vi "Select_User.vi"() -> ()   [LabVIEW 2016]
uses:
  <vilib>/Utility/miscctls.llb/LVPointTypeDef.ctl
  <vilib>/Utility/config.llb/NI_LVConfig.lvlib
panel:
  out "Controls references":T1
  out "GoToTracker indicator for Latching inside Events workaround":bool
  out "TestComm indicator for Latching inside Events workaround":bool
  in  "Login tab":enum32{"Login", "Settings", "Manage users"}(tab)
  in  "Go to Tracker":bool
  in  "Select User":u16(ring) items=["Admin"]
  in  "Enter password":string
  in  "Jump to tracking":bool
  in  "Button cover":bool
  out "Comm. test results":bool
  in  "Test VISA Comms":bool
  in  "VISA":refnum<visa-resource-name>="Tracker"
  in  "Cancel Users Update":bool
  in  "Save Users":bool
  in  "... or add new one":string
  in  "Reset or create password":string
  in  "Select User for update":u16(ring) items=["Admin"]
  in  "Delete current user":bool
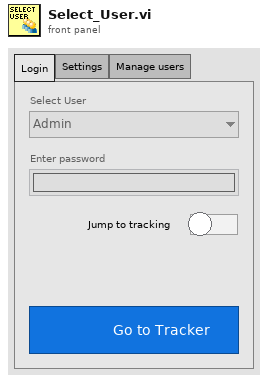
[diagram p1: front panel]
types:
  T1 = cluster{"Tabs":refnum<vi>, "Select User at login page":refnum<vi>, "Enter password":refnum<vi>, "Jump to tracking":refnum<vi>, "Test VISA Comms button":refnum<vi>, "Comm. test results indicator":refnum<vi>, "Select User for update":refnum<vi>, "Go to Tracker":refnum<vi>, "Jump to tracking":refnum<vi>, "... or add new one":refnum<vi>, "Reset or create password":refnum<vi>, "Delete current user":refnum<vi>}
  T2 = enum8{"Enabled", "Disabled", "Disabled and Grayed Out"}
  T3 = cluster{"Numeric Control":u32, "Numeric Control":u32}[]
  T4 = typedef "LVPointTypeDef.ctl" = cluster{"Horizontal":i16, "Vertical":i16}
  T5 = typedef "NI_LVConfig.lvlib/Config Data RefNum.ctl" = refnum<k1>
  T6 = typedef "eventvkey.ctl" = enum16{"ASCII", "Enter", "Return", "Shift", "Ctrl", "Alt", "Cmd", "Opt", "Caps", "NumLock", "Clear", "Break", "Up", "Down", "Left", "Right", "Insert", "Delete", "Home", "End", "PageUp", "PageDown", "Escape", "Help", "Pause", "ScrollLock", "F1", "F2", "F3", "F4", "F5", "F6", "F7", "F8", "F9", "F10", "F11", "F12", "F13", "F14", "F15", "F16", "F17", "F18", "F19", "F20", "F21", "F22", "F23", "F24", "Play", "VolumeUp", "VolumeDown", "Mute", "Two Byte Char"}
  T7 = enum32{"Page Enabled", "Page Disabled", "Page Disabled & Grayed"}
  T8 = cluster{"Data acquisition status":refnum<notifier>, "Play/Pause status":refnum<notifier>, "Complete stop":refnum<notifier>, "Temp file ready for processing":refnum<notifier>, "Has been recorded":refnum<notifier>, "Recording now":refnum<notifier>, "Path to the latest complete temp file":refnum<notifier>}
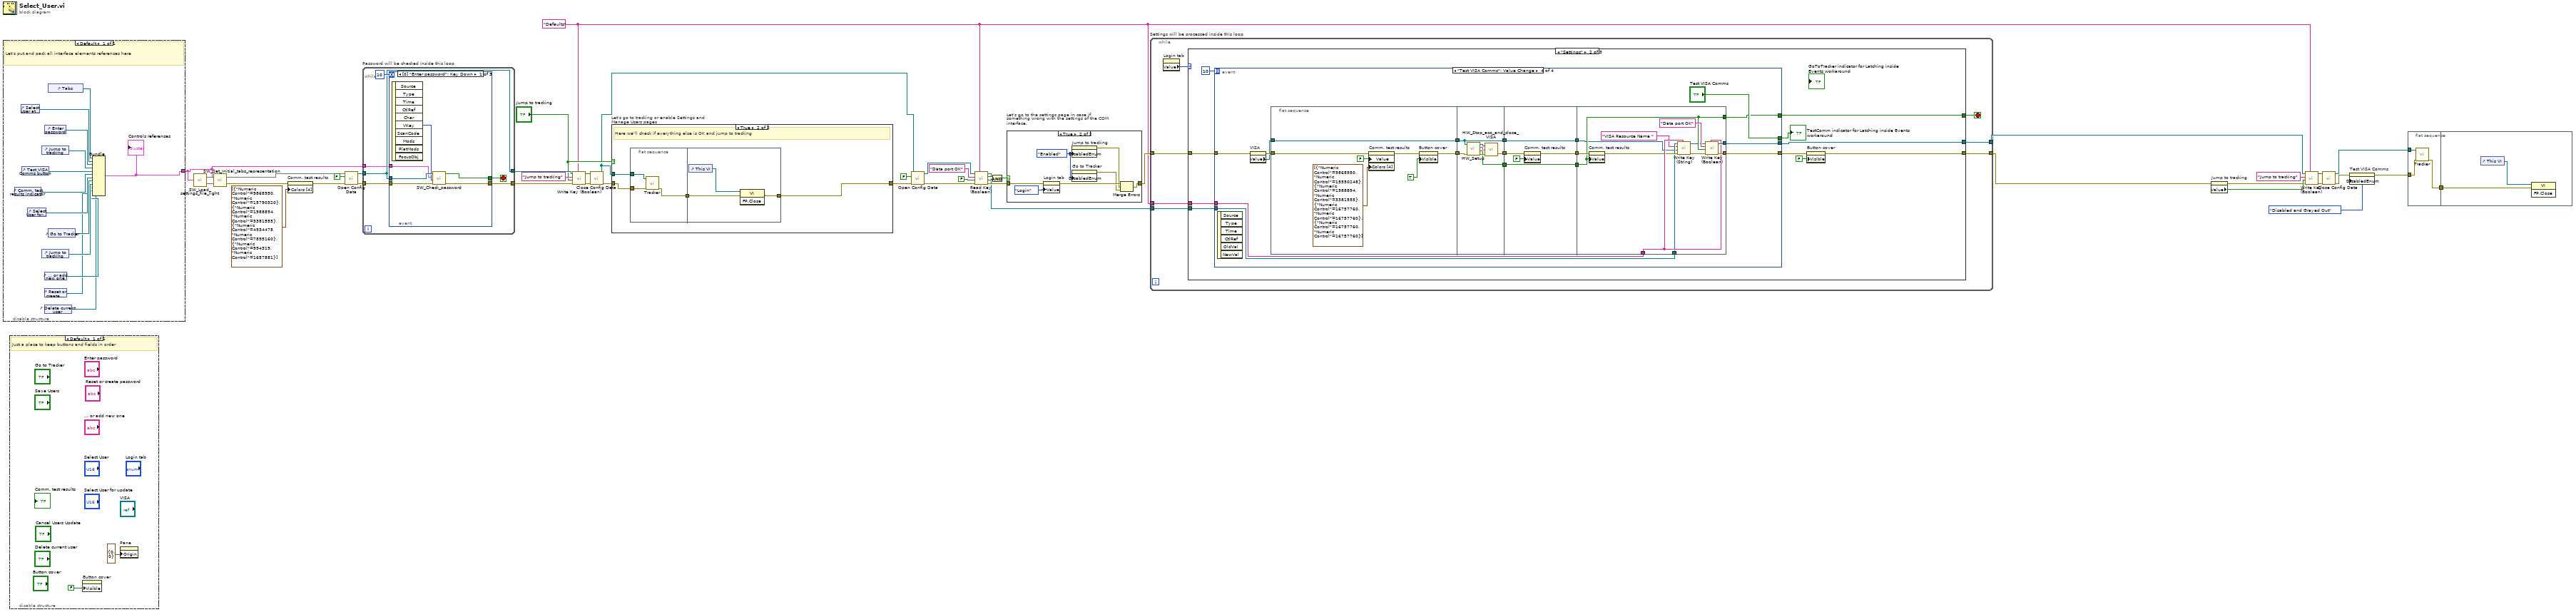
[diagram p0: block diagram]
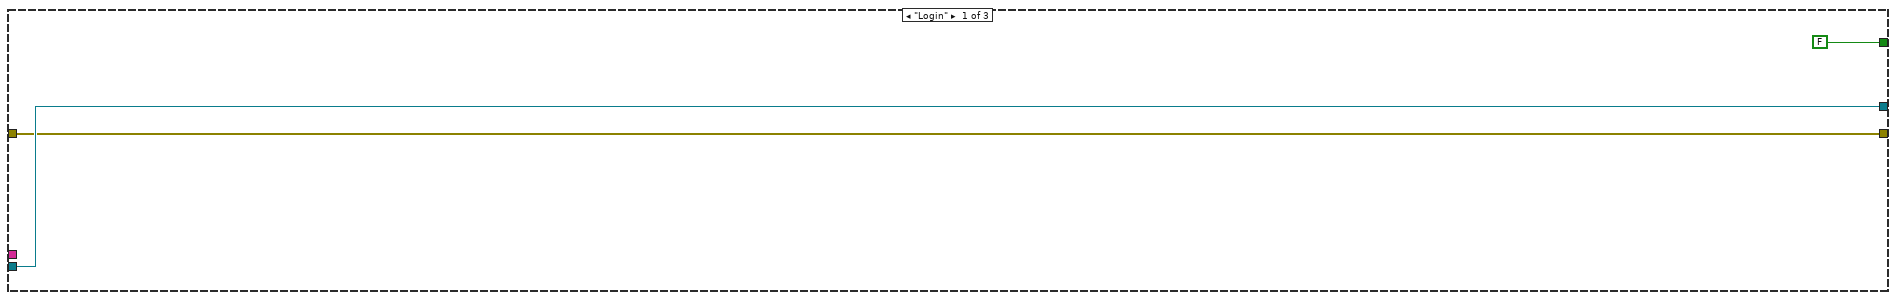
[diagram p2: hidden frame]
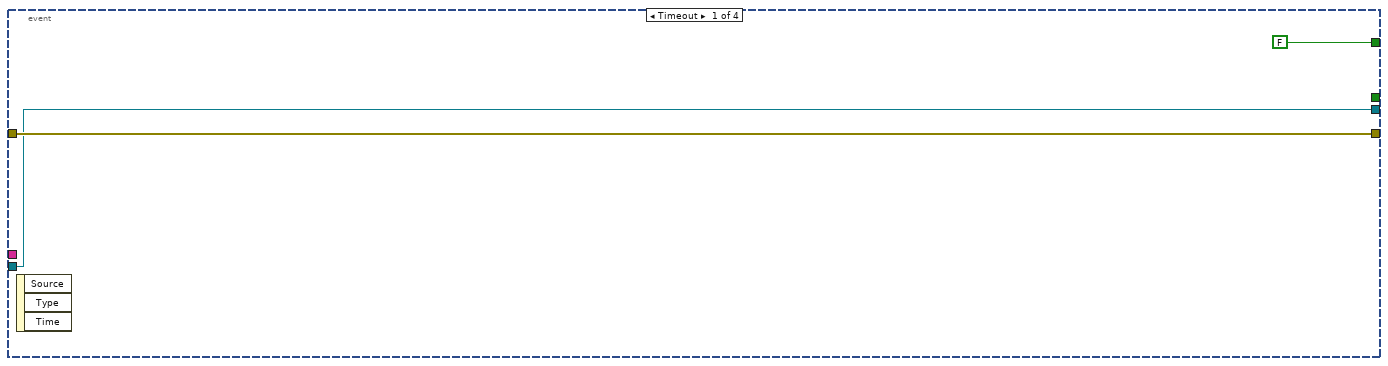
[diagram p3: hidden frame]
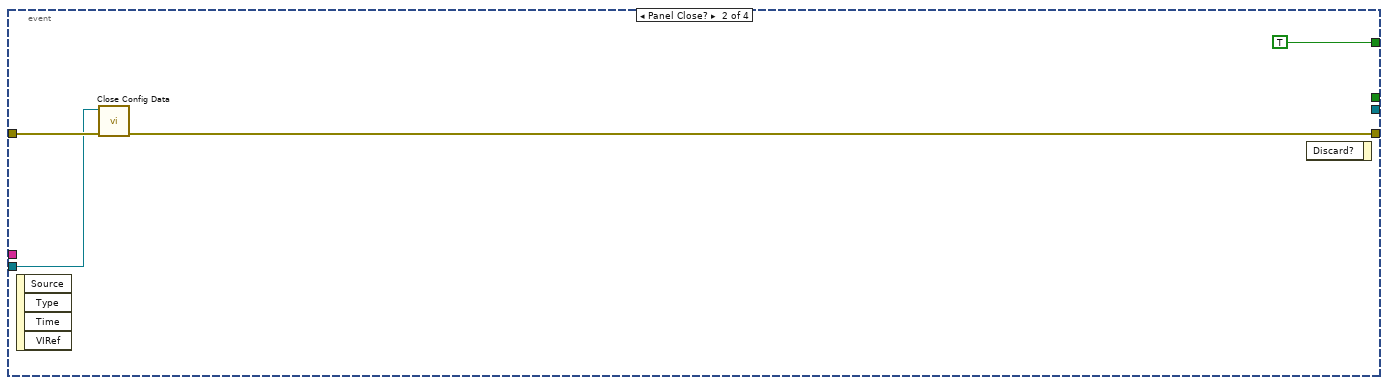
[diagram p4: hidden frame]
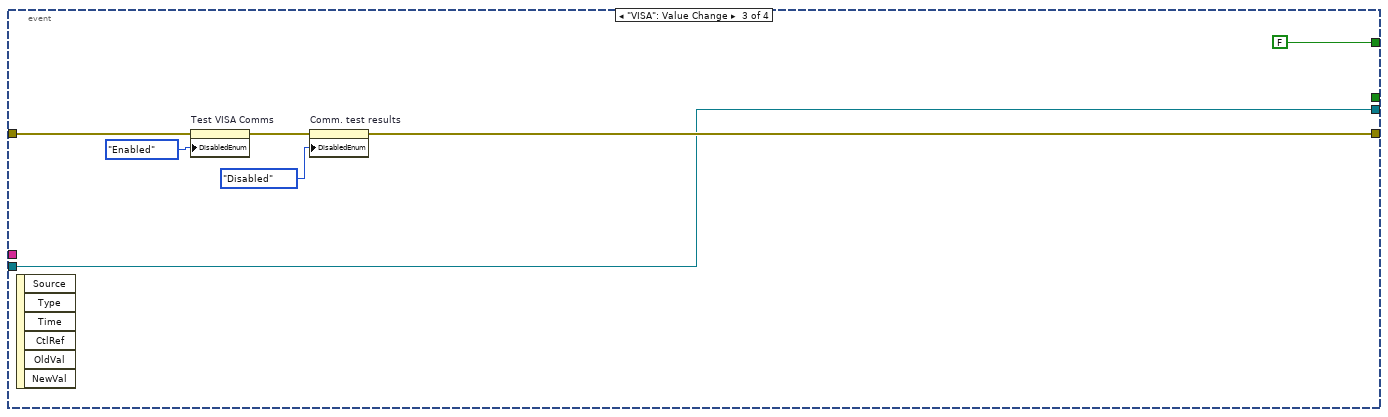
[diagram p5: hidden frame]
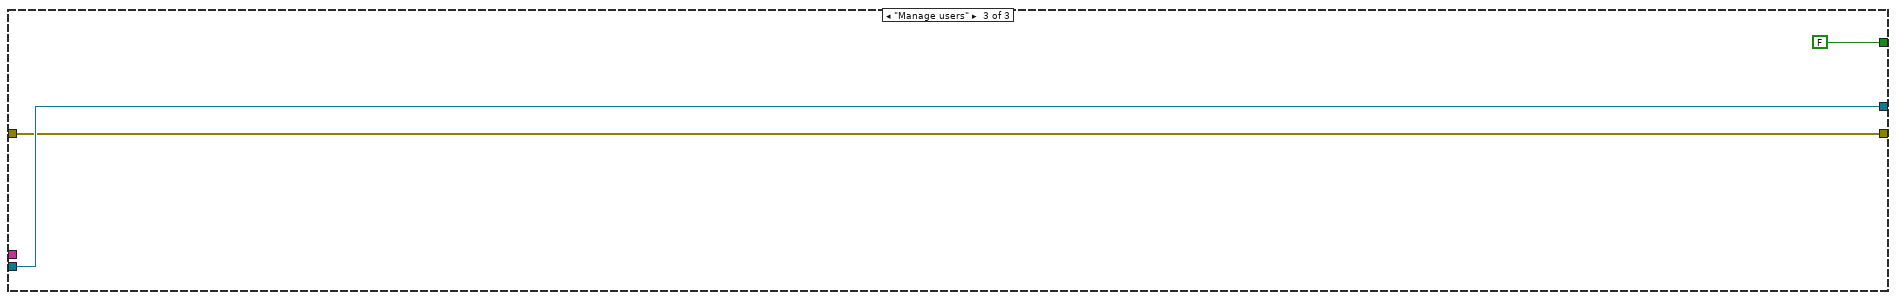
[diagram p6: hidden frame]
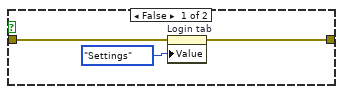
[diagram p7: hidden frame]
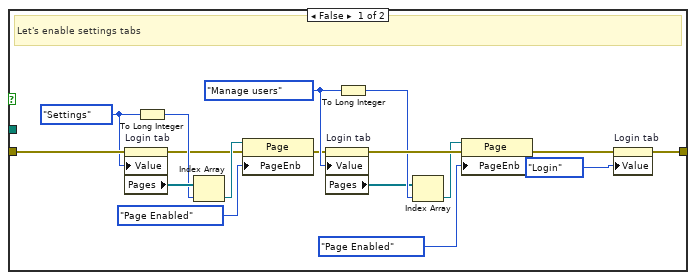
[diagram p8: hidden frame]
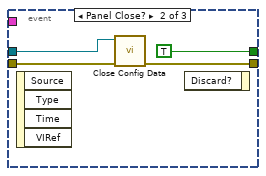
[diagram p9: hidden frame]
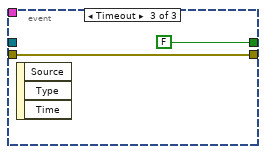
[diagram p10: hidden frame]
diagram:
  w9 = "Defaults" ("section")
  n1 = disable-structure "Conditional Disable Structure" shown="Default" {
    disable-tunnel: [w43] -> w3
    frame Enabled {
      # "Let's put and pack all interface elements references here"
      n2 = control-ref of="Comm. test results indicator"() -> (w50:refnum<vi>)
      n3 = control-ref of="Select User at login page"() -> (w54:refnum<vi>)
      n4 = control-ref of="Test VISA Comms button"() -> (w51:refnum<vi>)
      n5 = control-ref of="Select User for update"() -> (w49:refnum<vi>)
      n6 = control-ref of="Jump to tracking"() -> (w52:refnum<vi>)
      n7 = control-ref of="Jump to tracking"() -> (w47:refnum<vi>)
      n8 = control-ref of="Enter password"() -> (w53:refnum<vi>)
      n9 = control-ref of="... or add new one"() -> (w46:refnum<vi>)
      n10 = control-ref of="Reset or create password"() -> (w45:refnum<vi>)
      n11 = control-ref of="Delete current user"() -> (w44:refnum<vi>)
      n12 = control-ref of="Tabs"() -> (w55:refnum<vi>)
      n13 = control-ref of="Go to Tracker"() -> (w48:refnum<vi>)
      n14 = Bundle("Tabs"=w55, "Select User at login page"=w54, "Enter password"=w53, "Jump to tracking"=w52, "Test VISA Comms button"=w51, "Comm. test results indicator"=w50, "Select User for update"=w49, "Go to Tracker"=w48, "Jump to tracking"=w47, "... or add new one"=w46, "Reset or create password"=w45, "Delete current user"=w44) -> (w43:T1)  [unwired: 1 in]
      "Controls references" <- w43
    }
  }
  n15 = disable-structure shown="Default" {
    frame Enabled {
      # "Just a place to keep buttons and fields in order"
      n16 = property on="Button cover" class="Bool"("Visible"=FALSE) -> ()  [unwired: 2 in, 2 out]
      n17 = property on="Pane" class="Pane"("Origin"=T4 {"Horizontal"=0, "Vertical"=0}) -> ()  [unwired: 2 in, 2 out]
    }
  }
  n18 = call "SW_Load_settings_file_light.vi"(0:w3) -> (1:w22, 2:w40)
  n19 = call "SW_Set_Initial_tabs_representation.vi"("error in (no error)"=w40, "Controls references"=w3) -> ("error out"=w18:errorcluster)  [unwired: 1 in]
  n20 = property on="Comm. test results" class="Bool (strict)"(error in=w18, "Colors [4]"=T3 [{"Numeric Control"=9868950, "Numeric Control"=15790320}, {"Numeric Control"=1988894, "Numeric Control"=3381555}, {"Numeric Control"=4934475, "Numeric Control"=7895160}, {"Numeric Control"=994319, "Numeric Control"=1657881}]) -> (error out=w19:errorcluster)  [unwired: 1 in, 1 out]
  n21 = call <vilib>:"Open Config Data.vi"("error in (no error)"=w19, "create file if necessary (T)"=FALSE, "configuration file path"=w22) -> ("error out"=w41:errorcluster, "refnum"=w42:T5)  [unwired: 6 in, 1 out]
  n22 = while "Password will be checked inside this loop" {
    tunnel: w41 -> [w62]
    tunnel: w42 -> [w60]
    tunnel: [w61] -> w38
    tunnel: [w60] -> w39
    tunnel: w3 -> [w58]
    stop <- w59 stop-if-true
    n23 = event shown="[0] \"Enter password\": Key Down" {
      selector: _ -> [_ _ _]
      dyn-events: _ -> [_ _ _]
      timeout: 10 -> [_ _ _]
      tunnel: w62 -> [w69 w72 w74]
      tunnel: w60 -> [w68 w70 _]
      tunnel: [w66 TRUE ("Stop the loop") FALSE] -> w59
      tunnel: [w65 w71 w74] -> w61
      tunnel: w58 -> [w64 _ _]
      event "Enter password": Key Down {
        n24 = event-data() -> ("VKey"=w67:T6)  [unwired: 1 in, 9 out]
        n25 = call "SW_Check_password.vi"("error in (no error)"=w69, "Entered key"=w67, "Controls references"=w64, "Configuration file refnum in"=w68) -> ("error out"=w65:errorcluster, "Password OK"=w66:bool)  [unwired: 5 in, 1 out]
      }
      event Panel Close? {
        n26 = event-data() -> ()  [unwired: 1 in, 4 out]
        n27 = call <vilib>:"Close Config Data.vi"("error in (no error)"=w72, "refnum"=w70) -> ("error out"=w71:errorcluster)  [unwired: 8 in, 1 out]
        n28 = event-data() -> ()  [unwired: 2 in, 1 out]
      }
      event Timeout {
        n29 = event-data() -> ()  [unwired: 1 in, 3 out]
      }
    }
  }
  n30 = call <vilib>:"Write Key (Boolean).vi"("section"=w9, "error in (no error)"=w38, "value"="Jump to tracking", "key"="Jump to tracking", "refnum"=w39) -> ("error out"=w30:errorcluster, "refnum out"=w28:T5)  [unwired: 4 in, 1 out]
  n31 = call <vilib>:"Close Config Data.vi"("error in (no error)"=w30, "refnum"=w28) -> ("error out"=w29:errorcluster, "file path"=w1:path)  [unwired: 8 in]
  n32 = case "Let's go to tracking or enable Settings and Manage Users pages" shown="True" "Jump to tracking" {
    tunnel: w29 -> [w92 w96]
    tunnel: [w77 w93] -> w27
    tunnel: w1 -> [_ w95]
    frame False {
      w81 = enum32{"Login", "Settings", "Manage users"}."Manage users" ("Login tab")
      w90 = enum32{"Login", "Settings", "Manage users"}."Settings" ("Login tab")
      # "Let's enable settings tabs"
      n33 = property on="Login tab" class="TabCtl (strict)"(error in=w92, "Value"=w90) -> (error out=w87:errorcluster, "Pages"=w91:refnum<vi>[])  [unwired: 1 in, 1 out]
      n34 = To Long Integer(number=w90) -> (32bit integer=w89:i32)
      n35 = Index Array(array=w91, index=w89) -> (element=w88:refnum<vi>)
      n36 = property class="Page"(reference=w88, error in=w87, "PageEnb"=T7."Page Enabled" ("Page Enabled State")) -> (error out=w79:errorcluster)  [unwired: 1 out]
      n37 = property on="Login tab" class="TabCtl (strict)"(error in=w79, "Value"=w81) -> (error out=w84:errorcluster, "Pages"=w80:refnum<vi>[])  [unwired: 1 in, 1 out]
      n38 = To Long Integer(number=w81) -> (32bit integer=w82:i32)
      n39 = Index Array(array=w80, index=w82) -> (element=w83:refnum<vi>)
      n40 = property class="Page"(reference=w83, error in=w84, "PageEnb"=T7."Page Enabled" ("Page Enabled State")) -> (error out=w78:errorcluster)  [unwired: 1 out]
      n41 = property on="Login tab" class="TabCtl (strict)"(error in=w78, "Value"=enum32{"Login", "Settings", "Manage users"}."Login" ("Login tab")) -> (error out=w77:errorcluster)  [unwired: 1 in, 1 out]
    }
    frame True {
      # "Here we'll check if everything else is OK and jump to tracking"
      n42 = flat-sequence {
        tunnel: w96 -> [w99]
        tunnel: w95 -> [w98]
        tunnel: [w97] -> w94
        tunnel: w94 -> [w101]
        tunnel: [w100] -> w93
        frame #0 {
          n43 = call "Tracker.vi"("error in (no error)"=w99, "Settings file path"=w98) -> ("error out"=w97:errorcluster)  [unwired: 9 in]
        }
        frame #1 {
          n44 = control-ref of="This VI"() -> (w102:refnum<vi>)
          n45 = invoke class="VI" method="FP.Close"(reference=w102, error in=w101) -> (error out=w100:errorcluster)  [unwired: 1 in, 2 out]
        }
      }
    }
  }
  n46 = call <vilib>:"Open Config Data.vi"("error in (no error)"=w27, "create file if necessary (T)"=FALSE, "configuration file path"=w1) -> ("error out"=w26:errorcluster, "refnum"=w25:T5)  [unwired: 6 in, 1 out]
  n47 = call <vilib>:"Read Key (Boolean).vi"("section"=w9, "error in (no error)"=w26, "default value"=FALSE, "key"="Data port OK", "refnum"=w25) -> ("error out"=w31:errorcluster, "value"=w33:bool, "found?"=w34:bool, "refnum out"=w20:T5)  [unwired: 3 in]
  n48 = And(x=w34, y=w33) -> (x .and. y?=w32:bool)
  n49 = case "Let's go to the settings page in case if something wrong with the settings of the COM interface." shown="True" w32 {
    tunnel: w31 -> [w103 w112]
    tunnel: [w105 w109] -> w21
    frame False {
      n50 = property on="Login tab" class="TabCtl (strict)"(error in=w103, "Value"=enum32{"Login", "Settings", "Manage users"}."Settings" ("Login tab")) -> (error out=w105:errorcluster)  [unwired: 1 in, 1 out]
    }
    frame True {
      w110 = T2."Enabled" ("Disabled")
      n51 = property on="Login tab" class="TabCtl (strict)"(error in=w112, "Value"=enum32{"Login", "Settings", "Manage users"}."Login" ("Login tab")) -> (error out=w108:errorcluster)  [unwired: 1 in, 1 out]
      n52 = property on="Jump to tracking" class="Bool (strict)"("DisabledEnum"=w110) -> (error out=w107:errorcluster)  [unwired: 2 in, 1 out]
      n53 = property on="Go to Tracker" class="Bool"("DisabledEnum"=w110) -> (error out=w106:errorcluster)  [unwired: 2 in, 1 out]
      n54 = Merge Errors(w108, w107, w106) -> (w109:errorcluster)
    }
  }
  n55 = while "Settings will be processed inside this loop" {
    tunnel: w21 -> [w119]
    tunnel: w20 -> [w115]
    tunnel: [w117] -> w15
    tunnel: [w116] -> w14
    tunnel: w9 -> [w114]
    stop <- w118 stop-if-true
    n56 = property on="Login tab" class="TabCtl (strict)"() -> ("Value"=w113:enum32{"Login", "Settings", "Manage users"})  [unwired: 2 in, 2 out]
    n57 = case shown="\"Settings\"" w113 {
      tunnel: w119 -> [w121 w131 w196]
      tunnel: [FALSE ("Instrument OK?") w130 FALSE ("Instrument OK?")] -> w118
      tunnel: [w121 w126 w196] -> w117
      tunnel: [w122 w125 w197] -> w116
      tunnel: w115 -> [w122 w124 w197]
      tunnel: w114 -> [_ w123 _]
      frame "Login" {
      }
      frame "Settings" {
        n58 = event shown="[3] \"Test VISA Comms\": Value Change" {
          selector: _ -> [_ _ _ _]
          dyn-events: _ -> [_ _ _ _]
          timeout: 10 -> [_ _ _ _]
          tunnel: [w135 w137 w142 w158] -> w127
          tunnel: w131 -> [w135 w138 w146 w163]
          tunnel: [FALSE TRUE FALSE w149] -> w130
          tunnel: [_ _ _ "Test VISA Comms"] -> w129
          tunnel: [w133 _ w140 w151] -> w125
          tunnel: w124 -> [w133 w136 w140 w150]
          tunnel: w123 -> [_ _ _ w152]
          event Timeout {
            n59 = event-data() -> ()  [unwired: 1 in, 3 out]
          }
          event Panel Close? {
            n60 = event-data() -> ()  [unwired: 1 in, 4 out]
            n61 = call <vilib>:"Close Config Data.vi"("error in (no error)"=w138, "refnum"=w136) -> ("error out"=w137:errorcluster)  [unwired: 8 in, 1 out]
            n62 = event-data() -> ()  [unwired: 2 in, 1 out]
          }
          event "VISA": Value Change {
            n63 = event-data() -> ()  [unwired: 1 in, 6 out]
            n64 = property on="Test VISA Comms" class="Bool"(error in=w146, "DisabledEnum"=T2."Enabled" ("Disabled")) -> (error out=w145:errorcluster)  [unwired: 1 in, 1 out]
            n65 = property on="Comm. test results" class="Bool (strict)"(error in=w145, "DisabledEnum"=T2."Disabled" ("Disabled")) -> (error out=w142:errorcluster)  [unwired: 1 in, 1 out]
          }
          event "Test VISA Comms": Value Change {
            n66 = event-data() -> ()  [unwired: 1 in, 6 out]
            n67 = property on="VISA" class="VISAName"(error in=w163) -> (error out=w162:errorcluster, "Value"=w161:refnum<visa-resource-name>)  [unwired: 1 in, 1 out]
            n68 = flat-sequence {
              tunnel: w162 -> [w168]
              tunnel: w161 -> [w170]
              tunnel: [w170] -> w160
              tunnel: [w164] -> w159
              tunnel: w160 -> [w171]
              tunnel: w159 -> [w173]
              tunnel: [w174] -> w154
              tunnel: [w172] -> w156
              tunnel: [w171] -> w148
              tunnel: w156 -> [w179]
              tunnel: [w181] -> w155
              tunnel: w154 -> [w180]
              tunnel: [w180] -> w153
              tunnel: w148 -> [w178]
              tunnel: [w178] -> w147
              tunnel: [w192] -> w158
              tunnel: w155 -> [w194]
              tunnel: w153 -> [w190]
              tunnel: w152 -> [w189]
              tunnel: [w191] -> w151
              tunnel: w150 -> [w186]
              tunnel: [w190] -> w149
              tunnel: w147 -> [w184]
              frame #0 {
                n69 = property on="Comm. test results" class="Bool (strict)"(error in=w168, "Value"=FALSE ("Comm. test results"), "Colors [4]"=T3 [{"Numeric Control"=9868950, "Numeric Control"=15550248}, {"Numeric Control"=1988894, "Numeric Control"=3381555}, {"Numeric Control"=16757760, "Numeric Control"=16757760}, {"Numeric Control"=16757760, "Numeric Control"=16757760}]) -> (error out=w165:errorcluster)  [unwired: 1 in, 1 out]
                n70 = property on="Button cover" class="Bool"(error in=w165, "Visible"=TRUE) -> (error out=w164:errorcluster)  [unwired: 1 in, 1 out]
              }
              frame #1 {
                n71 = call "HW_Setup.vi"("VISA resource name in"=w171, "error in"=w173) -> ("VISA resource name out"=w177:refnum<visa-resource-name>, "Data flow controls"=w176:T8, "Instrument OK?"=w174:bool, "error out"=w175:errorcluster)  [unwired: 3 in, 1 out]
                n72 = call "HW_Stop_acq_and_close_VISA.vi"("error in"=w175, "Data flow controls in"=w176, "VISA resource name in"=w177) -> ("error out"=w172:errorcluster)  [unwired: 1 out]
              }
              frame #2 {
                n73 = property on="Comm. test results" class="Bool (strict)"(error in=w179, "Value"=FALSE ("Comm. test results")) -> (error out=w181:errorcluster)  [unwired: 1 in, 1 out]
              }
              frame #3 {
                n74 = property on="Comm. test results" class="Bool (strict)"(error in=w194, "Value"=w190) -> (error out=w187:errorcluster)  [unwired: 1 in, 1 out]
                n75 = call <vilib>:"Write Key (String).vi"("section"=w189, "error in (no error)"=w187, "value"=w184, "key"="VISA Resource Name ", "refnum"=w186) -> ("error out"=w188:errorcluster, "refnum out"=w185:T5)  [unwired: 4 in, 1 out]
                n76 = call <vilib>:"Write Key (Boolean).vi"("section"=w189, "error in (no error)"=w188, "value"=w190, "key"="Data port OK", "refnum"=w185) -> ("error out"=w192:errorcluster, "refnum out"=w191:T5)  [unwired: 4 in, 1 out]
              }
            }
          }
        }
        "TestComm indicator for Latching inside Events workaround" <- w129
        n77 = property on="Button cover" class="Bool"(error in=w127, "Visible"=FALSE) -> (error out=w126:errorcluster)  [unwired: 1 in, 1 out]
      }
      frame "Manage users" {
      }
    }
  }
  n78 = property on="Jump to tracking" class="Bool (strict)"(error in=w15) -> (error out=w12:errorcluster, "Value"=w13:bool)  [unwired: 1 in, 1 out]
  n79 = call <vilib>:"Write Key (Boolean).vi"("section"=w9, "error in (no error)"=w12, "value"=w13, "key"="Jump to tracking", "refnum"=w14) -> ("error out"=w11:errorcluster, "refnum out"=w10:T5)  [unwired: 4 in, 1 out]
  n80 = call <vilib>:"Close Config Data.vi"("error in (no error)"=w11, "refnum"=w10) -> ("error out"=w7:errorcluster, "file path"=w2:path)  [unwired: 8 in]
  n81 = property on="Test VISA Comms" class="Bool"(error in=w7, "DisabledEnum"=T2."Disabled and Grayed Out" ("Disabled")) -> (error out=w5:errorcluster)  [unwired: 1 in, 1 out]
  n82 = flat-sequence {
    tunnel: w5 -> [w200]
    tunnel: [w199] -> w4
    tunnel: w2 -> [w198]
    tunnel: w4 -> [w201]
    frame #0 {
      n83 = call "Tracker.vi"("error in (no error)"=w200, "Settings file path"=w198) -> ("error out"=w199:errorcluster)  [unwired: 9 in]
    }
    frame #1 {
      n84 = control-ref of="This VI"() -> (w202:refnum<vi>)
      n85 = invoke class="VI" method="FP.Close"(reference=w202, error in=w201) -> ()  [unwired: 1 in, 3 out]
    }
  }
